vi "qc5psm1.vi"() -> ()   [LabVIEW 2020]
uses:
  <instrlib>/CAEN PSM/CAEN PSM.lvlib
panel:
  in  "Tab Control":enum32{"Page 1"}(tab)
  in  "VISA resource name":refnum<visa-resource-name>
  in  "Voltage ramp up (0 V/s)":u16 max=999
  in  "Voltage Max (0.0 V)":u16=3000 max=9999
  in  "Board Address":i8 max=31
  in  "Vset":dbl
  out "OVV 2":bool
  out "OVC 2":bool
  out "V monitor 2":dbl(graph)
  out "I monitor 2":dbl(graph)
  out "R calc 2":dbl
  out "Actual current level (Imon)":dbl
  out "Actual voltage level (Vmon)":dbl
  in  "START AGAIN":bool
  out "Channel Status Array":T1(array[cluster])
  in  "Channel (0)":u8
  in  "Req (Mohm)":dbl=4.14
  out "TRIP":bool
  out "STATUS":string
  in  "CLOSE":bool
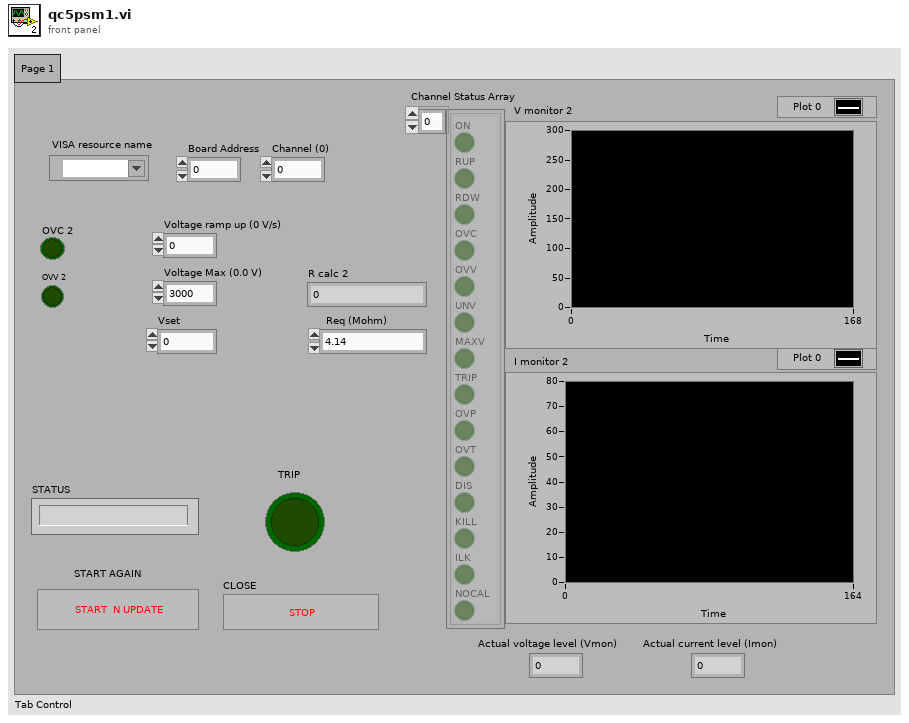
[diagram p1: front panel]
types:
  T1 = cluster{"ON":bool, "RUP":bool, "RDW":bool, "OVC":bool, "OVV":bool, "UNV":bool, "MAXV":bool, "TRIP":bool, "OVP":bool, "OVT":bool, "DIS":bool, "KILL":bool, "ILK":bool, "NOCAL":bool}[]
  T2 = cluster{"Baud Rate":u32, "Parity":enum16{"None", "Odd", "Even", "Mark", "Space"}, "Data Bits":u16, "Stop Bits":u16, "Flow Control":u16}
  T3 = typedef "CAEN PSM.lvlib/BoardHandle.ctl" = cluster{"VISA resource name":refnum<visa-resource-name>, "Board address":i8, "NChannels":u8}
  T4 = cluster{"ON":bool, "RUP":bool, "RDW":bool, "OVC":bool, "OVV":bool, "UNV":bool, "MAXV":bool, "TRIP":bool, "OVP":bool, "OVT":bool, "DIS":bool, "KILL":bool, "ILK":bool, "NOCAL":bool}
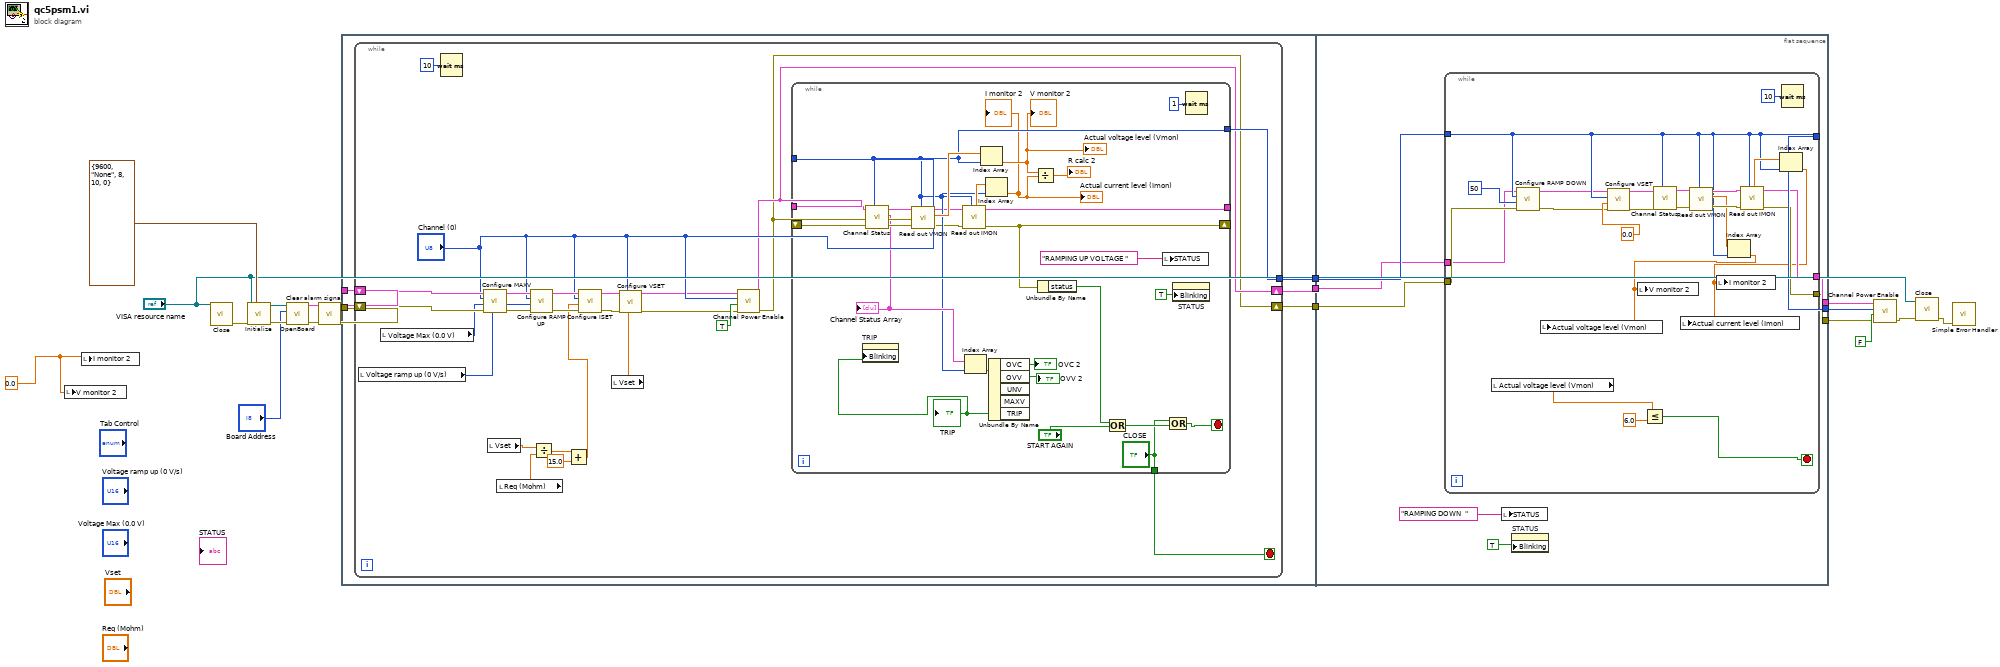
[diagram p0: block diagram]
diagram:
  w1 = 0.0
  n1 = local write "V monitor 2"(w1) -> ()
  n2 = local write "I monitor 2"(w1) -> ()
  n3 = call <instrlib>:"Close.vi"("VISA resource name"="VISA resource name") -> ("error out"=w12:errorcluster)  [unwired: 10 in]
  n4 = call <instrlib>:"Initialize.vi"("Serial Configuration"=T2 {"Baud Rate"=9600, "Parity"=enum."None", "Data Bits"=8, "Stop Bits"=10, "Flow Control"=0}, "error in (no error)"=w12, "VISA resource name"="VISA resource name") -> ("error out"=w19:errorcluster, "VISA resource name out"=w18:refnum<visa-resource-name>)  [unwired: 7 in]
  n5 = call <instrlib>:"OpenBoard.vi"("error in (no error)"=w19, "Board Address"="Board Address", "VISA resource name"=w18) -> ("error out"=w16:errorcluster, "BoardHandle"=w17:T3)  [unwired: 7 in]
  n6 = call <instrlib>:"Clear alarm signal.vi"("error in (no error)"=w16, "BoardHandle"=w17) -> ("error out"=w10:errorcluster, "BoardHandle out"=w11:T3)  [unwired: 8 in]
  n7 = flat-sequence {
    tunnel: w11 -> [w23]
    tunnel: w10 -> [w22]
    tunnel: [w25] -> w7
    tunnel: [w24] -> w6
    tunnel: [w21] -> w5
    tunnel: w7 -> [w78]
    tunnel: w6 -> [w85]
    tunnel: w5 -> [w84]
    tunnel: [w83] -> w4
    tunnel: [w82] -> w3
    tunnel: [w81] -> w2
    frame #0 {
      n8 = while {
        tunnel: [w50] -> w24
        shift-right: [w30] -> w25
        shift-left: w23 -> [w49]
        shift-right: [w29] -> w21
        shift-left: w22 -> [w48]
        stop <- w26 stop-if-true
        n9 = local read "Voltage ramp up (0 V/s)"() -> (w44:u16)
        n10 = local read "Voltage Max (0.0 V)"() -> (w45:u16)
        n11 = Wait (ms)(milliseconds to wait=u32 10) -> ()  [unwired: 1 out]
        n12 = call <instrlib>:"Configure MAXV.vi"("error in (no error)"=w48, "Voltage Max (0.0 V)"=w45, "Channel (0)"="Channel (0)", "BoardHandle"=w49) -> ("error out"=w46:errorcluster, "BoardHandle out"=w47:T3)  [unwired: 6 in]
        n13 = local read "Vset"() -> (w35:dbl)
        n14 = local read "Req (Mohm)"() -> (w34:dbl)
        n15 = call <instrlib>:"Configure RAMP UP.vi"("error in (no error)"=w46, "Voltage ramp up (0 V/s)"=w44, "Channel (0)"="Channel (0)", "BoardHandle"=w47) -> ("error out"=w40:errorcluster, "BoardHandle out"=w42:T3)  [unwired: 6 in]
        n16 = Divide(x=w35, y=w34) -> (x/y=w37:dbl)
        n17 = Add(x=w37, y=15.0) -> (x+y=w33:dbl)
        n18 = call <instrlib>:"Configure ISET.vi"("error in (no error)"=w40, "Current Limit (0.00 uA)"=w33, "Channel (0)"="Channel (0)", "BoardHandle"=w42) -> ("error out"=w39:errorcluster, "BoardHandle out"=w41:T3)  [unwired: 6 in]
        n19 = local read "Vset"() -> (w38:dbl)
        n20 = call <instrlib>:"Configure VSET.vi"("error in (no error)"=w39, "Voltage Level (0.0 V)"=w38, "Channel (0)"="Channel (0)", "BoardHandle"=w41) -> ("error out"=w27:errorcluster, "BoardHandle out"=w28:T3)  [unwired: 6 in]
        n21 = call <instrlib>:"Channel Power Enable.vi"("error in (no error)"=w27, "Enable (OFF)"=TRUE, "Channel (0)"="Channel (0)", "BoardHandle"=w28) -> ("error out"=w29:errorcluster, "BoardHandle out"=w30:T3)  [unwired: 6 in]
        n22 = while {
          shift-right: [w62] -> _
          shift-left: w29 -> [w63]
          tunnel: [w61] -> _
          tunnel: [w69] -> w50
          tunnel: w30 -> [w64]
          tunnel: "Channel (0)" -> [w69]
          tunnel: ["CLOSE"] -> w26
          stop <- w53 stop-if-true
          n23 = call <instrlib>:"Channel Status.vi"("Channel"=w69, "error in (no error)"=w63, "BoardHandle"=w64) -> ("error out"=w59:errorcluster, "Channel Status Array"=w76:T1, "BoardHandle out"=w60:T3)  [unwired: 5 in, 1 out]
          "Channel Status Array" <- w76
          n24 = call <instrlib>:"Read out VMON.vi"("Channel"=w69, "error in (no error)"=w59, "BoardHandle"=w60) -> ("error out"=w57:errorcluster, "VMon values (V)"=w77:dbl[], "BoardHandle out"=w58:T3)  [unwired: 6 in]
          n25 = call <instrlib>:"Read out IMON.vi"("Channel"=w69, "error in (no error)"=w57, "BoardHandle"=w58) -> ("error out"=w62:errorcluster, "IMon values (uA)"=w70:dbl[], "BoardHandle out"=w61:T3)  [unwired: 5 in, 1 out]
          n26 = Index Array(array=w76, index=w69) -> (element=w75:T4)
          n27 = Index Array(array=w77, index=w69) -> (element=w68:dbl)
          "Actual voltage level (Vmon)" <- w68
          "V monitor 2" <- w68
          n28 = Index Array(array=w70, index=w69) -> (element=w67:dbl)
          "Actual current level (Imon)" <- w67
          "I monitor 2" <- w67
          n29 = Unbundle By Name(w75) -> ("OVC"=→"OVC 2":bool, "OVV"=→"OVV 2":bool, "TRIP"=w56:bool)  [unwired: 2 out]
          "TRIP" <- w56
          n30 = property on="TRIP" class="Bool (strict)"("Blinking"=w56) -> ()  [unwired: 2 in, 2 out]
          n31 = Divide(x=w68, y=w67) -> (x/y=→"R calc 2":dbl)
          n32 = Unbundle By Name(w62) -> ("status"=w72:bool)
          n33 = Compound Arithmetic op=OR(w72, "START AGAIN") -> (w52:bool)
          n34 = local write "STATUS"("RAMPING UP VOLTAGE " ("String")) -> ()
          n35 = Compound Arithmetic op=OR("CLOSE", w52) -> (w53:bool)
          n36 = property on="STATUS" class="Str"("Blinking"=TRUE) -> ()  [unwired: 2 in, 2 out]
          n37 = Wait (ms)(milliseconds to wait=u32 1) -> ()  [unwired: 1 out]
        }
      }
    }
    frame #1 {
      n38 = while {
        tunnel: w85 -> [w95]
        tunnel: w84 -> [w107]
        tunnel: [w95] -> w83
        tunnel: [w98] -> w82
        tunnel: [w97] -> w81
        tunnel: w78 -> [w89]
        stop <- w92 stop-if-true
        n39 = local read "Actual voltage level (Vmon)"() -> (w86:dbl)
        n40 = call <instrlib>:"Configure RAMP DOWN.vi"("error in (no error)"=w107, "Voltage ramp down (0 V/s)"=u16 50, "Channel (0)"=w95, "BoardHandle"=w89) -> ("error out"=w87:errorcluster, "BoardHandle out"=w88:T3)  [unwired: 6 in]
        n41 = call <instrlib>:"Configure VSET.vi"("error in (no error)"=w87, "Voltage Level (0.0 V)"=0.0, "Channel (0)"=w95, "BoardHandle"=w88) -> ("error out"=w99:errorcluster, "BoardHandle out"=w96:T3)  [unwired: 6 in]
        n42 = Less Or Equal?(x=w86, y=6.0) -> (x <= y?=w92:bool)
        n43 = call <instrlib>:"Channel Status.vi"("Channel"=w95, "error in (no error)"=w99, "BoardHandle"=w96) -> ("error out"=w103:errorcluster, "BoardHandle out"=w102:T3)  [unwired: 5 in, 2 out]
        n44 = call <instrlib>:"Read out VMON.vi"("Channel"=w95, "error in (no error)"=w103, "BoardHandle"=w102) -> ("error out"=w105:errorcluster, "VMon values (V)"=w100:dbl[], "BoardHandle out"=w104:T3)  [unwired: 6 in]
        n45 = Index Array(array=w100, index=w95) -> (element=w94:dbl)
        n46 = local write "Actual voltage level (Vmon)"(w94) -> ()
        n47 = local write "V monitor 2"(w94) -> ()
        n48 = call <instrlib>:"Read out IMON.vi"("Channel"=w95, "error in (no error)"=w105, "BoardHandle"=w104) -> ("error out"=w97:errorcluster, "IMon values (uA)"=w101:dbl[], "BoardHandle out"=w98:T3)  [unwired: 5 in, 1 out]
        n49 = Index Array(array=w101, index=w95) -> (element=w93:dbl)
        n50 = local write "Actual current level (Imon)"(w93) -> ()
        n51 = local write "I monitor 2"(w93) -> ()
        n52 = Wait (ms)(milliseconds to wait=u32 10) -> ()  [unwired: 1 out]
      }
      n53 = local write "STATUS"("RAMPING DOWN  " ("String")) -> ()
      n54 = property on="STATUS" class="Str"("Blinking"=TRUE) -> ()  [unwired: 2 in, 2 out]
    }
  }
  n55 = call <instrlib>:"Channel Power Enable.vi"("error in (no error)"=w2, "Enable (OFF)"=FALSE, "Channel (0)"=w4, "BoardHandle"=w3) -> ("error out"=w14:errorcluster)  [unwired: 6 in, 1 out]
  n56 = call <instrlib>:"Close.vi"("error in (no error)"=w14, "VISA resource name"="VISA resource name") -> ("error out"=w13:errorcluster)  [unwired: 9 in]
  n57 = call <vilib>:"Simple Error Handler.vi"("error in (no error)"=w13) -> ()  [unwired: 4 in, 5 out]
